vi "ir_rsl.vi"   [LabVIEW 2012, in "Testing.lvrbt"]
uses:
  Testing.lvrbt
  <vilib>/NXT/HiTechnic/HiTechnic Controls/HiTechnic Port.ctl
  <vilib>/NXT/Block Support/NXT_InputPort.ctl
  <vilib>/NXT/Block Support/NXT_ButtonSelector.ctl
  <vilib>/NXT/Dual Mode Library/Sensors/readNXTButton.vi
  <vilib>/NXT/Dual Mode Library/Waits/Wait_Num.vi
  <vilib>/NXT/Dual Mode Library/Display/drawNumber.vi
types:
  T1 = typedef "HiTechnic Port.ctl" = cluster{"Port":T2, "MUX Port":u8}
  T2 = typedef "NXT_InputPort.ctl" = u32
  T3 = typedef "NXT_ButtonSelector.ctl" = u16
  T4 = cluster{"Direction (0-9)":i16, "Signal Strength (Array)":u8[]}
  T5 = typedef "LVHSConnector.ctl" = refnum<class "BrickReference.lvclass">
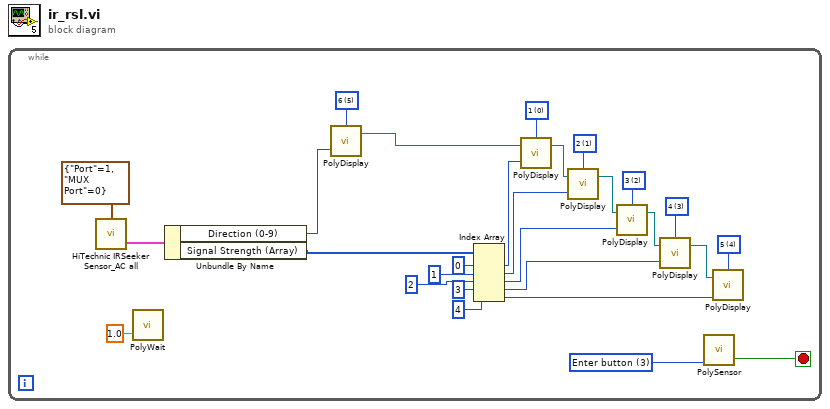
[diagram p0: block diagram]
diagram:
  n1 = while {
    stop <- w24 stop-if-true
    w11 = i16 4 items=["1", "2", "3", "4", "5", "6", "7", "8", "9", "10", "11", "12"] ("Line")
    w12 = i16 3 items=["1", "2", "3", "4", "5", "6", "7", "8", "9", "10", "11", "12"] ("Line")
    w13 = i16 2 items=["1", "2", "3", "4", "5", "6", "7", "8", "9", "10", "11", "12"] ("Line")
    w14 = i16 1 items=["1", "2", "3", "4", "5", "6", "7", "8", "9", "10", "11", "12"] ("Line")
    w19 = i16 0 items=["1", "2", "3", "4", "5", "6", "7", "8", "9", "10", "11", "12"] ("Line")
    w22 = i16 5 items=["1", "2", "3", "4", "5", "6", "7", "8", "9", "10", "11", "12"] ("Line")
    w25 = T3 3 items=["Enter button"=3, "Left button"=2, "Right button"=1, "Up Button"=4, "Down Button"=5] ("Button (Enter button)")
    n2 = call <vilib>:"HiTechnic IRSeeker Sensor_AC all.vi"("Port/MUX"=T1 {"Port"=1, "MUX Port"=0}) -> ("All Info"=w27:T4)  [unwired: 2 in, 1 out]
    n3 = call-poly <vilib>:"PolyWait.vi"("Time (1 sec)"=sgl 1.0) -> ()  [unwired: 3 in, 1 out]
    n4 = Unbundle By Name(w27) -> ("Direction (0-9)"=w21:i16, "Signal Strength (Array)"=w26:u8[])
    n5 = call-poly <vilib>:"PolyDisplay.vi"("number"=w21, "Line"=w22) -> ("NXT/EV3"=w5:T5)  [unwired: 2 in]
    n6 = Index Array(array=w26, index #1=0 ("index"), index #2=1 ("index"), index #3=2 ("index"), index #4=3 ("index"), index #5=4 ("index")) -> (element #1=w20:u8, element #2=w18:u8, element #3=w17:u8, element #4=w16:u8, element #5=w15:u8)
    n7 = call-poly <vilib>:"PolyDisplay.vi"("number"=w20, "NXT/EV3"=w5, "Line"=w19) -> ("NXT/EV3"=w4:T5)  [unwired: 1 in]
    n8 = call-poly <vilib>:"PolyDisplay.vi"("number"=w18, "NXT/EV3"=w4, "Line"=w14) -> ("NXT/EV3"=w3:T5)  [unwired: 1 in]
    n9 = call-poly <vilib>:"PolyDisplay.vi"("number"=w17, "NXT/EV3"=w3, "Line"=w13) -> ("NXT/EV3"=w2:T5)  [unwired: 1 in]
    n10 = call-poly <vilib>:"PolyDisplay.vi"("number"=w16, "NXT/EV3"=w2, "Line"=w12) -> ("NXT/EV3"=w1:T5)  [unwired: 1 in]
    n11 = call-poly <vilib>:"PolySensor.vi"("Button (Enter button)"=w25) -> ("Yes/No"=w24:bool)  [unwired: 2 in, 1 out]
    n12 = call-poly <vilib>:"PolyDisplay.vi"("number"=w15, "NXT/EV3"=w1, "Line"=w11) -> ()  [unwired: 1 in, 1 out]
  }
